vi "MENU_Internet.vi"(5 "FTP":bool=TRUE) -> (2 "FTP 2":bool=TRUE caption="FTP")   [LabVIEW 2010]
panel:
  in  "Close":bool
  # "FTP TRANSFER ON/OFF"
  # "No"
  # "Yes"
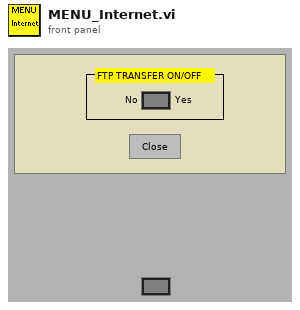
[diagram p1: front panel]
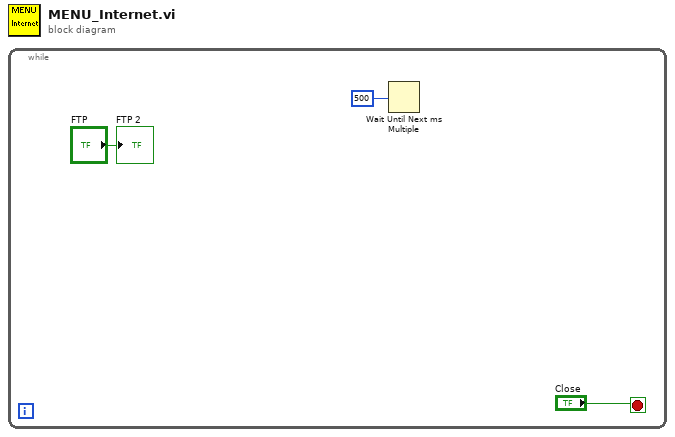
[diagram p0: block diagram]
diagram:
  n1 = while {
    stop <- "Close" stop-if-true
    n2 = Wait Until Next ms Multiple(millisecond multiple=500) -> ()  [unwired: 1 out]
    "FTP 2" <- "FTP"
  }
